vi "ErrorCode-MsgLookup.vi"(5 "DLL Return Code":i32) -> (0 "NI-DAQ Error Code":i32, 1 "DAQ Error?":bool, 2 "Error String":string)   [LabVIEW 2024]
uses:
  Program Files (x86)/Luna Technologies/OVA 5000 v5.14.2/data/OVA32.dll
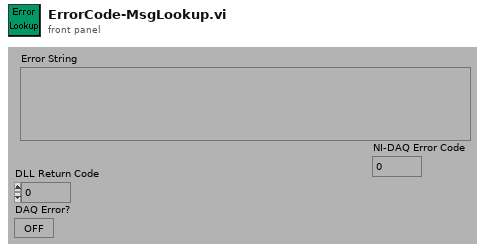
[diagram p1: front panel]
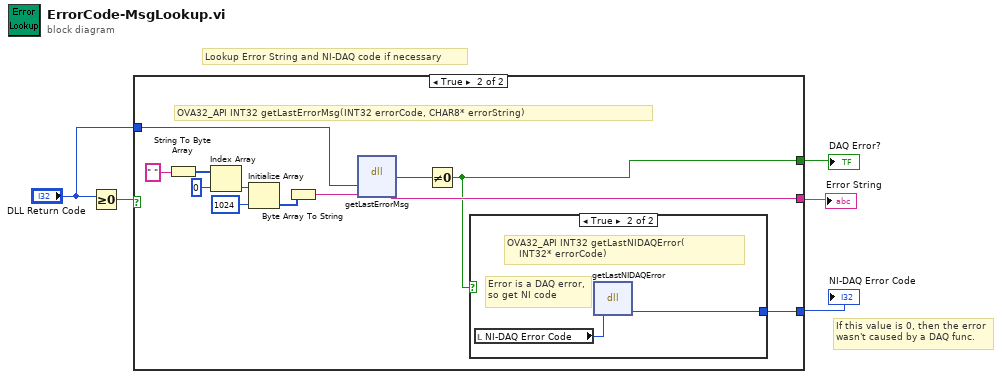
[diagram p0: block diagram]
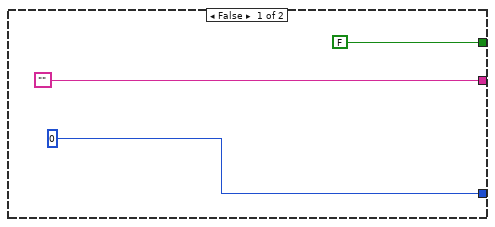
[diagram p2: hidden frame]
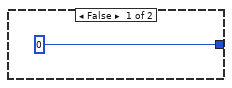
[diagram p3: hidden frame]
diagram:
  # "If this value is 0, then the error\nwasn't caused by a DAQ func."
  # "Lookup Error String and NI-DAQ code if necessary"
  n1 = Greater Or Equal To 0?(x="DLL Return Code") -> (x >= 0?=w1:bool)
  n2 = case shown="True" w1 {
    tunnel: ["" w13] -> w5
    tunnel: [0 ("errorCode") w10] -> w4
    tunnel: "DLL Return Code" -> [_ w12]
    tunnel: [FALSE w9] -> w3
    frame False {
    }
    frame True {
      # "OVA32_API INT32 getLastErrorMsg(INT32 errorCode, CHAR8* errorString)"
      n3 = String To Byte Array(string=" ") -> (unsigned byte array=w19:u8[])
      n4 = Index Array(array=w19, index=0 ("Index")) -> (element=w17:u8)
      n5 = Initialize Array(w17, 1024 ("Dimension Size")) -> (w15:u8[])
      n6 = Byte Array To String(unsigned byte array=w15) -> (string=w14:string)
      n7 = dll-call lib="C:/Program Files (x86)/Luna Technologies/OVA 5000 v5.14.2/data/OVA32.dll" fn="getLastErrorMsg"("errorCode_DLL"=w12, "errorMsg"=w14) -> ("return type"=w11:i32, "errorMsg"=w13:string)  [unwired: 4 in, 2 out]
      n8 = Not Equal To 0?(x=w11) -> (x != 0?=w9:bool)
      n9 = case shown="True" w9 {
        tunnel: [0 ("errorCode") w22] -> w10
        frame False {
        }
        frame True {
          # "OVA32_API INT32 getLastNIDAQError(\n    INT32* errorCode)"
          # "Error is a DAQ error,\nso get NI code"
          n10 = local read "NI-DAQ Error Code"() -> (w23:i32)
          n11 = dll-call lib="C:/Program Files (x86)/Luna Technologies/OVA 5000 v5.14.2/data/OVA32.dll" fn="getLastNIDAQError"("errorCode"=w23) -> ("errorCode"=w22:i32)  [unwired: 4 in, 2 out]
        }
      }
    }
  }
  "Error String" <- w5
  "NI-DAQ Error Code" <- w4
  "DAQ Error?" <- w3
